vi "Torque_calculation.vi"(10 "Position":dbl, 11 "speed":dbl) -> (3 "Torque":dbl)   [LabVIEW 2013]
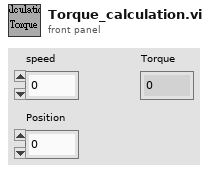
[diagram p1: front panel]
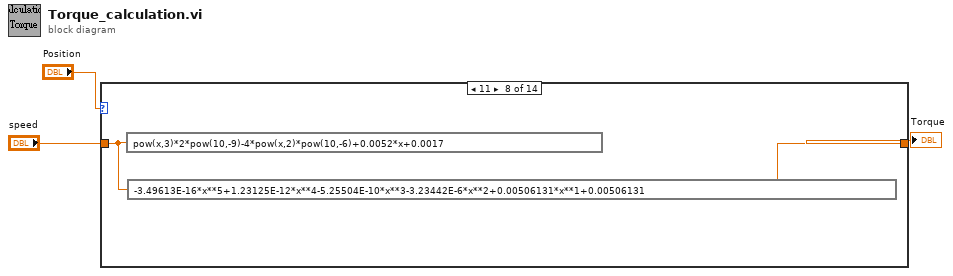
[diagram p0: block diagram]
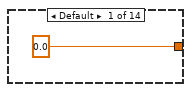
[diagram p2: hidden frame]
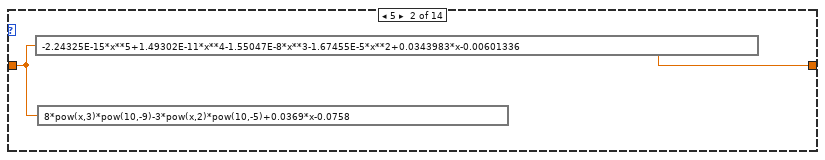
[diagram p3: hidden frame]
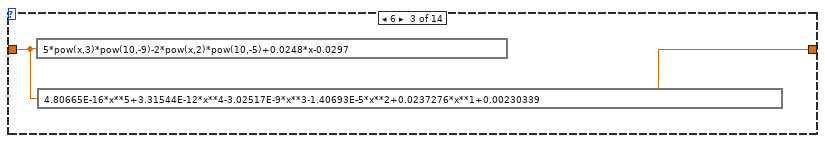
[diagram p4: hidden frame]
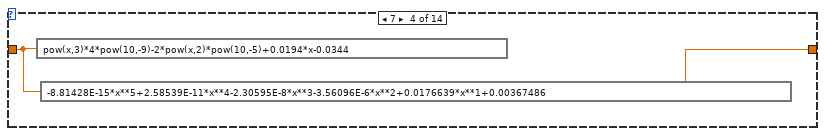
[diagram p5: hidden frame]
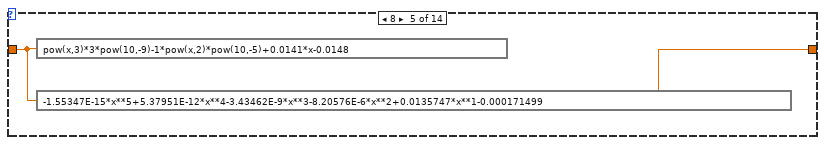
[diagram p6: hidden frame]
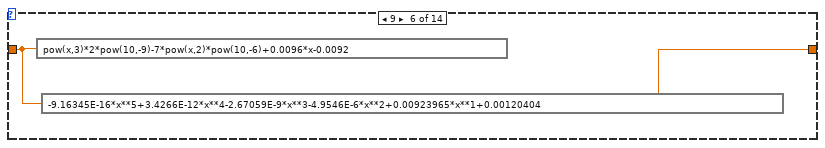
[diagram p7: hidden frame]
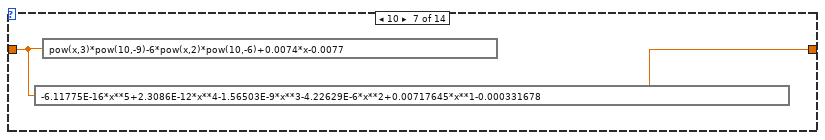
[diagram p8: hidden frame]
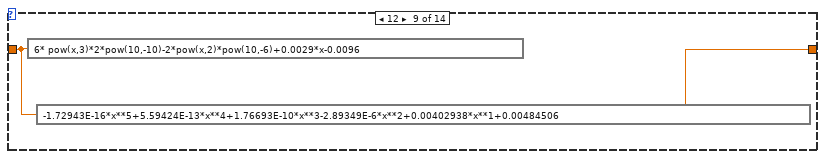
[diagram p9: hidden frame]
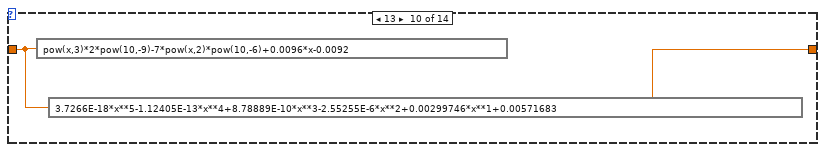
[diagram p10: hidden frame]
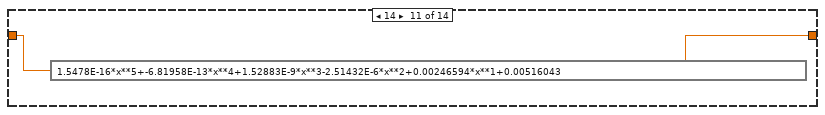
[diagram p11: hidden frame]
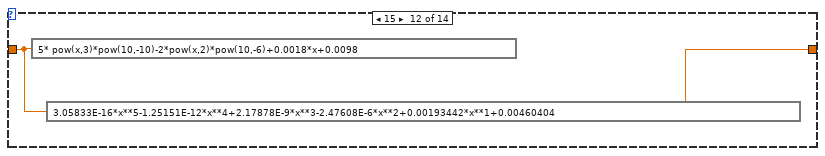
[diagram p12: hidden frame]
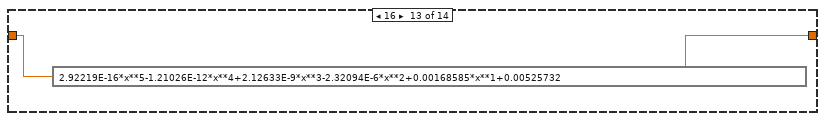
[diagram p13: hidden frame]
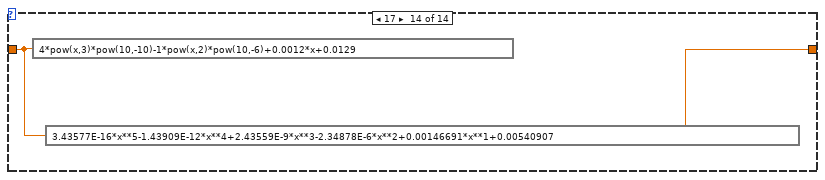
[diagram p14: hidden frame]
diagram:
  n1 = case shown="11" "Position" {
    tunnel: [0.0 ("speed") w5 w7 w9 w11 w13 w15 w17 w19 w21 w23 w25 w27 w29] -> w3
    tunnel: "speed" -> [_ w6 w8 w10 w12 w14 w16 w18 w20 w22 w24 w26 w28 w30]
    frame Default {
    }
    frame 5 {
      n2 = expression code="-2.24325E-15*x**5+1.49302E-11*x**4-1.55047E-8*x**3-1.67455E-5*x**2+0.0343983*x-0.00601336"(w6) -> (w5:dbl)
      n3 = expression code="8*pow(x,3)*pow(10,-9)-3*pow(x,2)*pow(10,-5)+0.0369*x-0.0758"(w6) -> ()  [unwired: 1 out]
    }
    frame 6 {
      n4 = expression code="5*pow(x,3)*pow(10,-9)-2*pow(x,2)*pow(10,-5)+0.0248*x-0.0297"(w8) -> ()  [unwired: 1 out]
      n5 = expression code="4.80665E-16*x**5+3.31544E-12*x**4-3.02517E-9*x**3-1.40693E-5*x**2+0.0237276*x**1+0.00230339"(w8) -> (w7:dbl)
    }
    frame 7 {
      n6 = expression code="pow(x,3)*4*pow(10,-9)-2*pow(x,2)*pow(10,-5)+0.0194*x-0.0344"(w10) -> ()  [unwired: 1 out]
      n7 = expression code="-8.81428E-15*x**5+2.58539E-11*x**4-2.30595E-8*x**3-3.56096E-6*x**2+0.0176639*x**1+0.00367486"(w10) -> (w9:dbl)
    }
    frame 8 {
      n8 = expression code="pow(x,3)*3*pow(10,-9)-1*pow(x,2)*pow(10,-5)+0.0141*x-0.0148"(w12) -> ()  [unwired: 1 out]
      n9 = expression code="-1.55347E-15*x**5+5.37951E-12*x**4-3.43462E-9*x**3-8.20576E-6*x**2+0.0135747*x**1-0.000171499"(w12) -> (w11:dbl)
    }
    frame 9 {
      n10 = expression code="pow(x,3)*2*pow(10,-9)-7*pow(x,2)*pow(10,-6)+0.0096*x-0.0092"(w14) -> ()  [unwired: 1 out]
      n11 = expression code="-9.16345E-16*x**5+3.4266E-12*x**4-2.67059E-9*x**3-4.9546E-6*x**2+0.00923965*x**1+0.00120404"(w14) -> (w13:dbl)
    }
    frame 10 {
      n12 = expression code="-6.11775E-16*x**5+2.3086E-12*x**4-1.56503E-9*x**3-4.22629E-6*x**2+0.00717645*x**1-0.000331678"(w16) -> (w15:dbl)
      n13 = expression code="pow(x,3)*pow(10,-9)-6*pow(x,2)*pow(10,-6)+0.0074*x-0.0077"(w16) -> ()  [unwired: 1 out]
    }
    frame 11 {
      n14 = expression code="pow(x,3)*2*pow(10,-9)-4*pow(x,2)*pow(10,-6)+0.0052*x+0.0017"(w18) -> ()  [unwired: 1 out]
      n15 = expression code="-3.49613E-16*x**5+1.23125E-12*x**4-5.25504E-10*x**3-3.23442E-6*x**2+0.00506131*x**1+0.00506131"(w18) -> (w17:dbl)
    }
    frame 12 {
      n16 = expression code="6* pow(x,3)*2*pow(10,-10)-2*pow(x,2)*pow(10,-6)+0.0029*x-0.0096"(w20) -> ()  [unwired: 1 out]
      n17 = expression code="-1.72943E-16*x**5+5.59424E-13*x**4+1.76693E-10*x**3-2.89349E-6*x**2+0.00402938*x**1+0.00484506"(w20) -> (w19:dbl)
    }
    frame 13 {
      n18 = expression code="pow(x,3)*2*pow(10,-9)-7*pow(x,2)*pow(10,-6)+0.0096*x-0.0092"(w22) -> ()  [unwired: 1 out]
      n19 = expression code="3.7266E-18*x**5-1.12405E-13*x**4+8.78889E-10*x**3-2.55255E-6*x**2+0.00299746*x**1+0.00571683"(w22) -> (w21:dbl)
    }
    frame 14 {
      n20 = expression code="1.5478E-16*x**5+-6.81958E-13*x**4+1.52883E-9*x**3-2.51432E-6*x**2+0.00246594*x**1+0.00516043"(w24) -> (w23:dbl)
    }
    frame 15 {
      n21 = expression code="5* pow(x,3)*pow(10,-10)-2*pow(x,2)*pow(10,-6)+0.0018*x+0.0098"(w26) -> ()  [unwired: 1 out]
      n22 = expression code="3.05833E-16*x**5-1.25151E-12*x**4+2.17878E-9*x**3-2.47608E-6*x**2+0.00193442*x**1+0.00460404"(w26) -> (w25:dbl)
    }
    frame 16 {
      n23 = expression code="2.92219E-16*x**5-1.21026E-12*x**4+2.12633E-9*x**3-2.32094E-6*x**2+0.00168585*x**1+0.00525732"(w28) -> (w27:dbl)
    }
    frame 17 {
      n24 = expression code="4*pow(x,3)*pow(10,-10)-1*pow(x,2)*pow(10,-6)+0.0012*x+0.0129"(w30) -> ()  [unwired: 1 out]
      n25 = expression code="3.43577E-16*x**5-1.43909E-12*x**4+2.43559E-9*x**3-2.34878E-6*x**2+0.00146691*x**1+0.00540907"(w30) -> (w29:dbl)
    }
  }
  "Torque" <- w3
